vi "Channels.Inline.Read.Channel Block Descriptor.vi"(8 "error in (no error)":errorcluster, 10 "Values Array in":dbl[](array[numeric]), 11 "Channel Block Descriptor":T1[](array[typedef])) -> (0 "error out":errorcluster, 2 "Values Array out":dbl[](array[numeric]), 3 "Channel Block Descriptor dup":T1[](array[typedef]))   [LabVIEW 2016, in "VeriStand Data.lvlib"]
doc: "Reads the block of channel data specified by <B>Channel Block Descriptor</B> into the provided <B>Values Array</B>."
uses:
  VeriStand Data.lvlib
  Typedefs/Typedefs.Block Descriptor.Channel Block.ctl
  Typedefs/Typedefs.Block Descriptor.ctl
  Memory Management/Memory Management.MoveByteBlock.Write (Double).vi
  Memory Management/Memory Management.Handle Return.vi
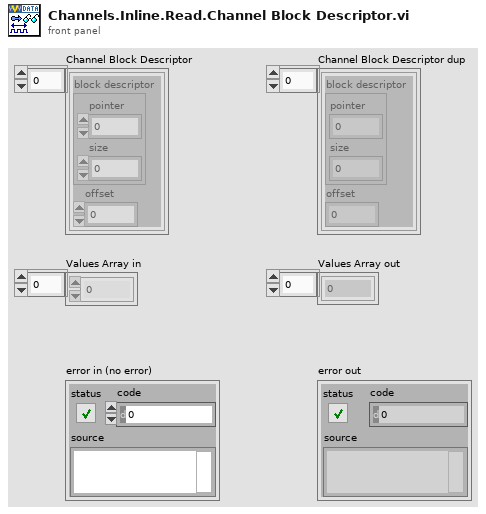
[diagram p1: front panel]
types:
  T1 = typedef "VeriStand Data.lvlib/Typedefs.Block Descriptor.Channel Block.ctl" = cluster{"block descriptor":T2, "offset":u64}
  T2 = typedef "VeriStand Data.lvlib/Typedefs.Block Descriptor.ctl" = cluster{"pointer":u64, "size":i64}
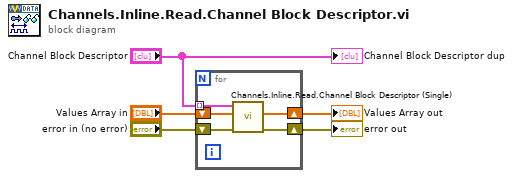
[diagram p0: block diagram]
diagram:
  n1 = for {
    shift-right: [w8] -> w3
    shift-left: "error in (no error)" -> [w10]
    shift-right: [w7] -> w2
    shift-left: "Values Array in" -> [w9]
    tunnel: "Channel Block Descriptor" -> [w6] mode=indexing
    n2 = call "Channels.Inline.Read.Channel Block Descriptor (Single).vi"("error in (no error)"=w10, "Values Array in"=w9, "Channel Block Descriptor"=w6) -> ("error out"=w8:errorcluster, "Values Array out"=w7:dbl[])  [unwired: 6 in, 1 out]
  }
  "Values Array out" <- w2
  "error out" <- w3
  "Channel Block Descriptor dup" <- "Channel Block Descriptor"
